vi "Stop Core.vi"(10 "final error code":i32, 11 "Form Server in":refnum<class "Form Server.lvclass">) -> (3 "Form Server out":refnum<class "Form Server.lvclass">)   [LabVIEW 2020]
doc: "(<B>Filename</B>: Actor Framework.lvlib:Actor.lvclass:Stop Core.vi)\n\nDefines what the actor does before it stops. Use the <B>final error code</B> input to determine whether the actor shut down in response to an error.\n\nBy default, this method passes the Stop message along to all auto-stop nested actors. A descendant class may override this method to define additional behavior, such as shutting down any processes the actor initiated in its override of the Actor Core method."
uses:
  Form Server.lvclass
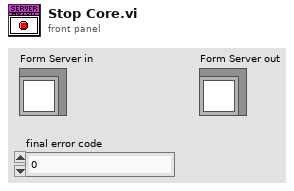
[diagram p1: front panel]
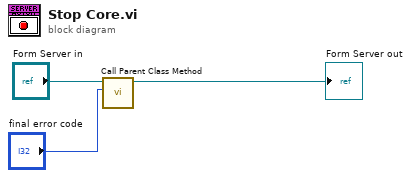
[diagram p0: block diagram]
diagram:
  n1 = call-parent "Call Parent Class Method"("final error code"="final error code", "Monitored Actor in"="Form Server in") -> ("Monitored Actor out"=→"Form Server out":refnum<class "Form Server.lvclass">)  [unwired: 9 in]
